vi "TestStand - End Modal Dialog.vi"(0 "Sequence Context In":T1, 5 "Modal ID":i32, 7 "VI Originally Open":bool, 11 "error in (no error)":errorcluster) -> (15 "error out":errorcluster)   [LabVIEW 2012]
doc: "Stops the calling dialog box VI from being modal to the TestStand main application window."
uses:
  6.0/DifferentStdPrototype/LabVIEW Test - Sequence Context.ctl
  user32.dll
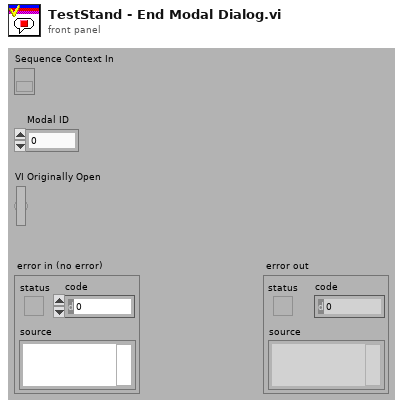
[diagram p1: front panel]
types:
  T1 = typedef "LabVIEW Test - Sequence Context.ctl" = refnum<k7>
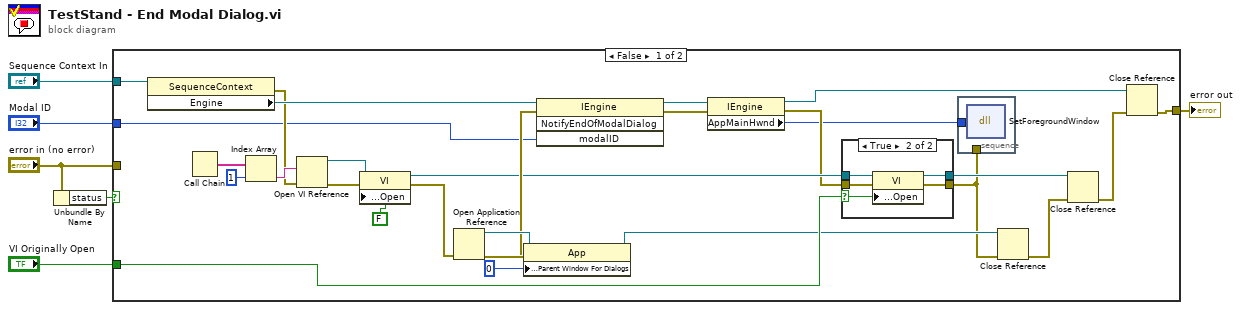
[diagram p0: block diagram]
diagram:
  n1 = Unbundle By Name("error in (no error)") -> ("status"=w3:bool)
  n2 = case shown="False" w3 {
    tunnel: "Sequence Context In" -> [w29 _]
    tunnel: [w22 w43] -> w5
    tunnel: "error in (no error)" -> [_ w43]
    tunnel: "Modal ID" -> [w17 _]
    tunnel: "VI Originally Open" -> [w16 _]
    frame False {
      n3 = property class="SequenceContext"(reference=w29) -> (error out=w27:errorcluster, "Engine"=w28:refnum<k7>)  [unwired: 1 in, 1 out]
      n4 = Call Chain() -> (call chain=w34:string[])
      n5 = Index Array(array=w34, index=1 ("Index")) -> (element=w32:string)
      n6 = Open VI Reference(vi path=w32, error in (no error)=w27) -> (vi reference=w30:refnum<vi>, error out=w31:errorcluster)  [unwired: 4 out]
      n7 = property class="VI"(reference=w30, error in=w31, "Front Panel Window:Open"=FALSE) -> (reference out=w15:refnum<vi>, error out=w20:errorcluster)
      n8 = Open Application Reference(8:w20) -> (0:w26:errorcluster, 3:w25:refnum<vi>)  [unwired: 3 out]
      n9 = property class="App"(reference=w25, error in=w26, "Application:Parent Window For Dialogs"=0) -> (reference out=w14:refnum<vi>, error out=w18:errorcluster)
      n10 = invoke class="IEngine" method="NotifyEndOfModalDialog"(reference=w28, error in=w18, "modalID"=w17) -> (reference out=w11:refnum<k7>, error out=w12:errorcluster)  [unwired: 1 in, 2 out]
      n11 = property class="IEngine"(reference=w11, error in=w12) -> (reference out=w9:refnum<k7>, error out=w10:errorcluster, "AppMainHwnd"=w8:i32)
      n12 = case shown="True" w16 {
        selector: w16 -> [_ w38]
        tunnel: [w37 w39] -> w7
        tunnel: w10 -> [w37 w42]
        tunnel: [w36 w40] -> w13
        tunnel: w15 -> [w36 w41]
        frame False {
        }
        frame True {
          n13 = property class="VI"(reference=w41, error in=w42, "Front Panel Window:Open"=w38) -> (reference out=w40:refnum<vi>, error out=w39:errorcluster)
        }
      }
      n14 = stacked-sequence {
        tunnel: w8 -> [w35]
        tunnel: w7 -> [_]
        frame #0 {
          n15 = dll-call lib="user32.dll" fn="SetForegroundWindow"("hWnd"=w35) -> ()  [unwired: 4 in, 3 out]
        }
      }
      n16 = Close Reference(reference=w14, error in (no error)=w7) -> (error out=w24:errorcluster)
      n17 = Close Reference(reference=w13, error in (no error)=w24) -> (error out=w23:errorcluster)
      n18 = Close Reference(reference=w9, error in (no error)=w23) -> (error out=w22:errorcluster)
    }
    frame True {
    }
  }
  "error out" <- w5
